vi "Instruments.vi"() -> ()   [LabVIEW 2016, in "Hall Effect Library.lvlib"]
uses:
  Hall Effect Library.lvlib
  Public/Controls/Ammeters.ctl
  Public/Controls/I-Sources.ctl
  Public/Controls/Voltmeters.ctl
  Public/Controls/Magnets.ctl
  Public/Controls/Switches.ctl
panel:
  in  "Switch":T1
  in  "Magnet":T2
  in  "Voltmeter":T3=enum."2182A"
  in  "Current Source":T4=enum."26XX"
  in  "Ammeter":T5=enum."648X"
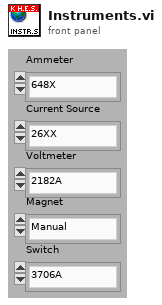
[diagram p1: front panel]
types:
  T1 = typedef "Hall Effect Library.lvlib/Switches.ctl" = enum16{"3706A"}
  T2 = typedef "Hall Effect Library.lvlib/Magnets.ctl" = enum16{"Manual"}
  T3 = typedef "Hall Effect Library.lvlib/Voltmeters.ctl" = enum16{"2000", "2182A", "3706A"}
  T4 = typedef "Hall Effect Library.lvlib/I-Sources.ctl" = enum16{"622X", "26XX"}
  T5 = typedef "Hall Effect Library.lvlib/Ammeters.ctl" = enum16{"None", "648X"}
diagram:
